vi "Launch Save Status.vi"(8 "error in":errorcluster, 10 "Status":string, 11 "Master Controller in":refnum<class "EMS User Interface.lvclass">) -> (0 "error out":errorcluster, 3 "Master Controller out":refnum<class "EMS User Interface.lvclass">)   [LabVIEW 2018, in "EMS User Interface Actor.lvlib" / "EMS User Interface.lvclass"]
uses:
  EMS User Interface.lvclass
  C:/Program Files (x86)/National Instruments/LabVIEW 2018/vi.lib/ActorFramework/Actor/Actor.lvclass
  C:/Users/Administrator/Desktop/2018LabVIEW EMS/EMS Generic Actor/EMS Generic/EMS Generic.lvclass
  Dialog Actors/Save File Actor/Save File/Save File.lvclass
  EMS Generic Actor/EMS Generic/EMS Generic.lvclass/EMS Generic.ctl
  Dialog Actors/Save File Actor/Save File/Save File.lvclass/Save File.ctl
  <vilib>/ActorFramework/Actor/Actor.lvclass
  EMS Generic Actor/EMS Generic/EMS Generic.lvclass
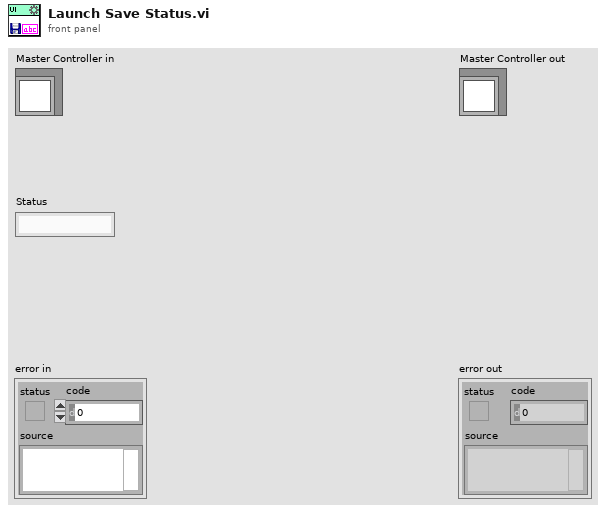
[diagram p1: front panel]
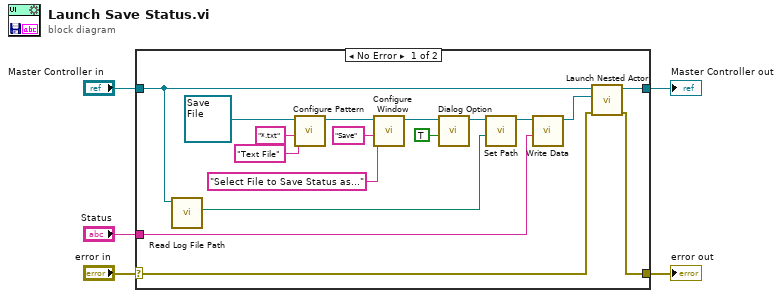
[diagram p0: block diagram]
diagram:
  n1 = case shown="No Error" "error in" {
    selector: "error in" -> [w9 w24]
    tunnel: [w8 w24] -> w4
    tunnel: [w11 w23] -> w2
    tunnel: "Master Controller in" -> [w7 w23]
    tunnel: "Status" -> [w12 _]
    frame No Error {
      n2 = call "Read Log File Path.vi"("EMS Generic in"=w7) -> ("Log File Path"=w6:path)  [unwired: 8 in, 2 out]
      n3 = call "Configure Pattern.vi"("Pattern Label"="Text File", "Pattern"="*.txt", "Save File in"=refnum<class "Save File.lvclass"> refnum) -> ("Save File out"=w19:refnum<class "Save File.lvclass">)  [unwired: 8 in]
      n4 = call "Configure Window.vi"("Prompt"="Select File to Save Status as...", "Button Label"="Save", "Save File in"=w19) -> ("Save File out"=w16:refnum<class "Save File.lvclass">)  [unwired: 8 in]
      n5 = call "Dialog Option.vi"("Dialog?"=TRUE, "Save File in"=w16) -> ("Save File out"=w14:refnum<class "Save File.lvclass">)  [unwired: 9 in]
      n6 = call "Set Path.vi"("Path"=w6, "Save File in"=w14) -> ("Save File out"=w13:refnum<class "Save File.lvclass">)  [unwired: 9 in]
      n7 = call "Write Data.vi"("Data"=w12, "Save File in"=w13) -> ("Save File out"=w10:refnum<class "Save File.lvclass">)  [unwired: 9 in]
      n8 = call <vilib>:"Launch Nested Actor.vi"("error in (no error)"=w9, "Nested Actor"=w10, "Caller Actor in"=w7) -> ("error out"=w8:errorcluster, "Caller Actor out"=w11:refnum<class "EMS User Interface.lvclass">)  [unwired: 6 in, 1 out]
    }
    frame Error {
    }
  }
  "error out" <- w4
  "Master Controller out" <- w2
